vi "Single Clothoid Calculation.vi"(9 "Angle":dbl, 10 "Min R":dbl) -> (3 "Zeroes out":T1)   [LabVIEW 2019]
uses:
  BlendType.ctl
  Globals.vi
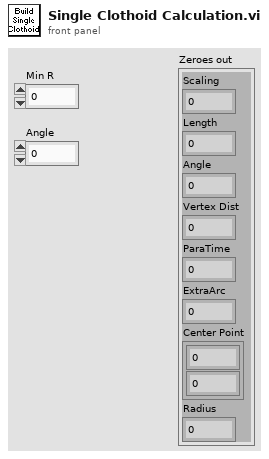
[diagram p1: front panel]
types:
  T1 = typedef "BlendType.ctl" = cluster{"Scaling":dbl, "Length":dbl, "Angle":dbl, "Vertex Dist":dbl, "ParaTime":dbl, "ExtraArc":dbl, "Center Point":cluster{dbl, dbl}, "Radius":dbl}
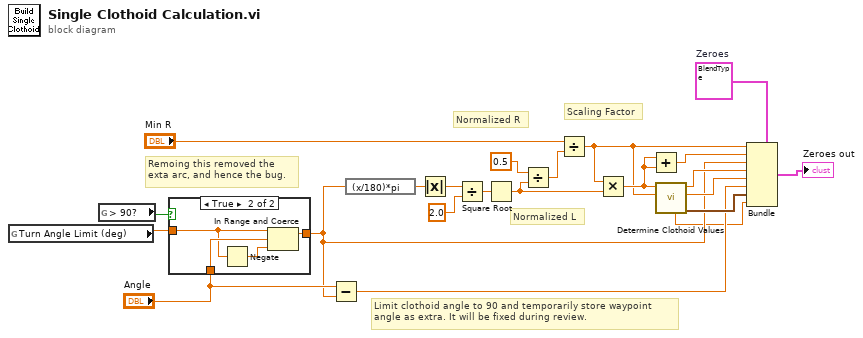
[diagram p0: block diagram]
diagram:
  w8 = T1 {"Scaling"=0.0, "Length"=0.0, "Angle"=0.0, "Vertex Dist"=0.0, "ParaTime"=0.0, "ExtraArc"=0.0, "Center Point"={0.0, 0.0}, "Radius"=0.0}  # Zeroes
  # "Remoing this removed the\nexta arc, and hence the bug."
  # "Limit clothoid angle to 90 and temporarily store waypoint\nangle as extra. It will be fixed during review."
  # "Normalized L"
  # "Scaling Factor"
  # "Normalized R"
  n1 = global read "Globals.vi" "Turn Angle Limit (deg)"() -> (w2:dbl)
  n2 = global read "Globals.vi" "> 90?"() -> (w3:bool)
  n3 = case shown="True" w3 {
    tunnel: "Angle" -> [w23 w27]
    tunnel: [w23 w26] -> w6
    tunnel: w2 -> [_ w24]
    frame False {
    }
    frame True {
      n4 = Negate(x=w24) -> (-x=w25:dbl)
      n5 = In Range and Coerce(upper limit=w24, x=w27, lower limit=w25) -> (coerced(x)=w26:dbl)  [unwired: 1 out]
    }
  }
  n6 = Subtract(x="Angle", y=w6) -> (x-y=w4:dbl)
  n7 = expression code="(x/180)*pi" ("radians to degrees")(w6) -> (w5:dbl)
  n8 = Absolute Value(x=w5) -> (abs(x)=w16:dbl)
  n9 = Divide(x=w16, y=2.0) -> (x/y=w12:dbl)
  n10 = Square Root(x=w12) -> (sqrt(x)=w21:dbl)
  n11 = Divide(x=0.5, y=w21) -> (x/y=w10:dbl)
  n12 = Divide(x="Min R", y=w10) -> (x/y=w18:dbl)
  n13 = Multiply(x=w18, y=w21) -> (x*y=w19:dbl)
  n14 = Add(x=w19, y=w19) -> (x+y=w20:dbl)
  n15 = call "Determine Clothoid Values.vi"("Scaling"=w18, "Desired Length"=w19) -> ("Center Point"=w22:cluster{dbl, dbl}, "Para Time"=w15:dbl, "Vertex Dist ft"=w17:dbl, "Radius"=w1:dbl)  [unwired: 5 in, 1 out]
  n16 = Bundle(cluster=w8, "Scaling"=w18, "Length"=w20, "Angle"=w6, "Vertex Dist"=w17, "ParaTime"=w15, "ExtraArc"=w4, "Center Point"=w22, "Radius"=w1) -> (→"Zeroes out":T1)
